vi "Get Tag Name.vi"(8 "error in (no error)":errorcluster, 11 "VI in":refnum<vi>) -> (0 "error out":errorcluster, 2 "String":string, 3 "VI out":refnum<vi>)   [LabVIEW 2021]
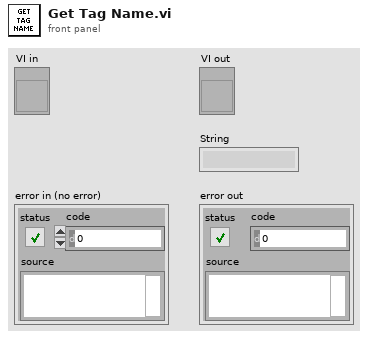
[diagram p1: front panel]
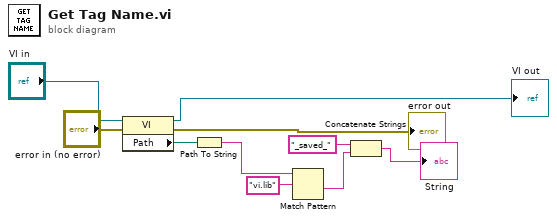
[diagram p0: block diagram]
diagram:
  n1 = property class="VI"(reference="VI in", error in="error in (no error)") -> (reference out=→"VI out":refnum<vi>, error out=→"error out":errorcluster, "Path"=w6:path)
  n2 = Path To String(path=w6) -> (string=w8:string)
  n3 = Match Pattern(string=w8, regular expression="vi.lib") -> (after substring=w9:string)  [unwired: 1 in, 3 out]
  n4 = Concatenate Strings("_saved_" ("string"), w9) -> (→"String":string)
